vi "DrawMoreFrame.vi"(1 "ROI":T1={"Global Rectangle"=[0, 0, 0, 0], "Contours"=[{"ID"=enum."External", "Type"=3, "Coordinates"=[0, 0, 0, 0]}]} {"Contours"."Type" items=["No Selection", "Point", "Line", "Rectangle", "Oval", "Polygon", "Free", "Annulus", "Unused2", "Unused3", "Broken Line", "Free Hand Line", "Rotated Rectangle"]}, 2 "Color":u32(colorbox)=16711680, 3 "Image Out 2":T4, 4 "MoreFram":i32[][](array[numeric]), 5 "Rect_Center":i32[](array[numeric]), 6 "Rect-Cluster":T3, 7 "MoreFrame":T2(array[cluster])) -> (0 "Image Out":T4)   [LabVIEW 2014]
uses:
  <vilib>/vision/Image Controls.llb/IMAQ Image.ctl
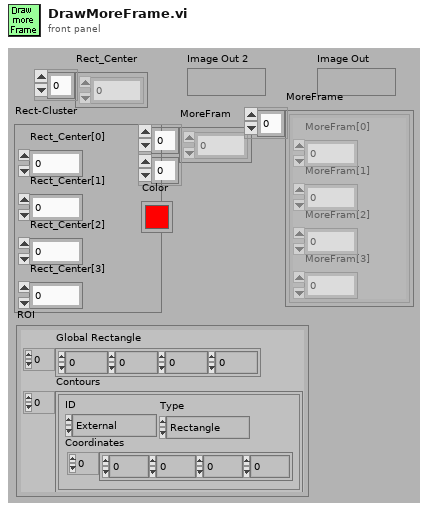
[diagram p1: front panel]
types:
  T1 = cluster{"Global Rectangle":i32[], "Contours":cluster{"ID":enum32{"External", "Internal"}, "Type":u32, "Coordinates":i32[]}[]}
  T2 = cluster{"MoreFram[0]":i32, "MoreFram[1]":i32, "MoreFram[2]":i32, "MoreFram[3]":i32}[]
  T3 = cluster{"Rect_Center[0]":i32, "Rect_Center[1]":i32, "Rect_Center[2]":i32, "Rect_Center[3]":i32}
  T4 = typedef "IMAQ Image.ctl" = refnum<image>
  T5 = cluster{"ID":enum32{"External", "Internal"}, "Type":u32, "Coordinates":i32[]}[]
  T6 = cluster{"ID":enum32{"External", "Internal"}, "Type":u32, "Coordinates":i32[]}
  T7 = cluster{"MoreFram[0]":i32, "MoreFram[1]":i32, "MoreFram[2]":i32, "MoreFram[3]":i32}
  T8 = cluster{"Coordinates[0]":i32, "Coordinates[1]":i32, "Coordinates[2]":i32, "Coordinates[3]":i32}
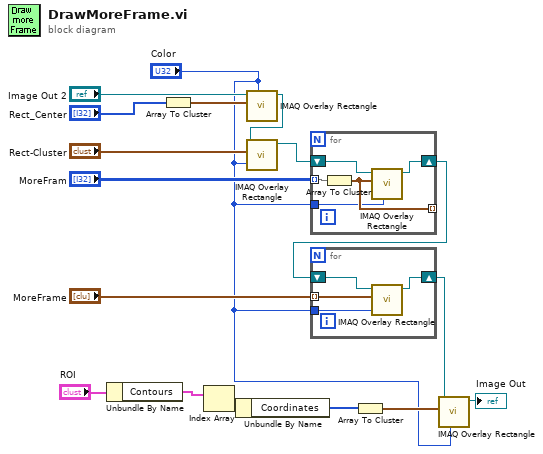
[diagram p0: block diagram]
diagram:
  n1 = Unbundle By Name("ROI") -> ("Contours"=w7:T5)
  n2 = Array To Cluster(array="Rect_Center") -> (cluster=w15:T3)
  n3 = Index Array(array=w7) -> (element=w6:T6)  [unwired: 1 in]
  n4 = Unbundle By Name(w6) -> ("Coordinates"=w4:i32[])
  n5 = call "IMAQ Overlay Rectangle"("Color"="Color", "Rectangle"=w15, "Image"="Image Out 2") -> ("Image Out"=w13:T4)  [unwired: 3 in, 5 out]
  n6 = call "IMAQ Overlay Rectangle"("Color"="Color", "Rectangle"="Rect-Cluster", "Image"=w13) -> ("Image Out"=w11:T4)  [unwired: 3 in, 5 out]
  n7 = for {
    tunnel: "MoreFram" -> [w22] mode=indexing
    shift-right: [w20] -> w10
    shift-left: w11 -> [w21]
    tunnel: [w19] -> _ mode=indexing
    tunnel: "Color" -> [w18]
    n8 = Array To Cluster(array=w22) -> (cluster=w19:T7)
    n9 = call "IMAQ Overlay Rectangle"("Color"=w18, "Rectangle"=w19, "Image"=w21) -> ("Image Out"=w20:T4)  [unwired: 3 in, 5 out]
  }
  n10 = for {
    shift-right: [w25] -> w3
    shift-left: w10 -> [w26]
    tunnel: "MoreFrame" -> [w24] mode=indexing
    tunnel: "Color" -> [w23]
    n11 = call "IMAQ Overlay Rectangle"("Color"=w23, "Rectangle"=w24, "Image"=w26) -> ("Image Out"=w25:T4)  [unwired: 3 in, 5 out]
  }
  n12 = Array To Cluster(array=w4) -> (cluster=w5:T8)
  n13 = call "IMAQ Overlay Rectangle"("Color"="Color", "Rectangle"=w5, "Image"=w3) -> ("Image Out"=→"Image Out":T4)  [unwired: 3 in, 5 out]
